vi "test_json_decode.vi"() -> (0 "error out":errorcluster, 3 "all_passed":bool)   [LabVIEW 2019]
panel:
  out "passed":bool[](array[boolean])
  out "values":T1(array[cluster])
  in  "test_cases":T2(array[cluster])
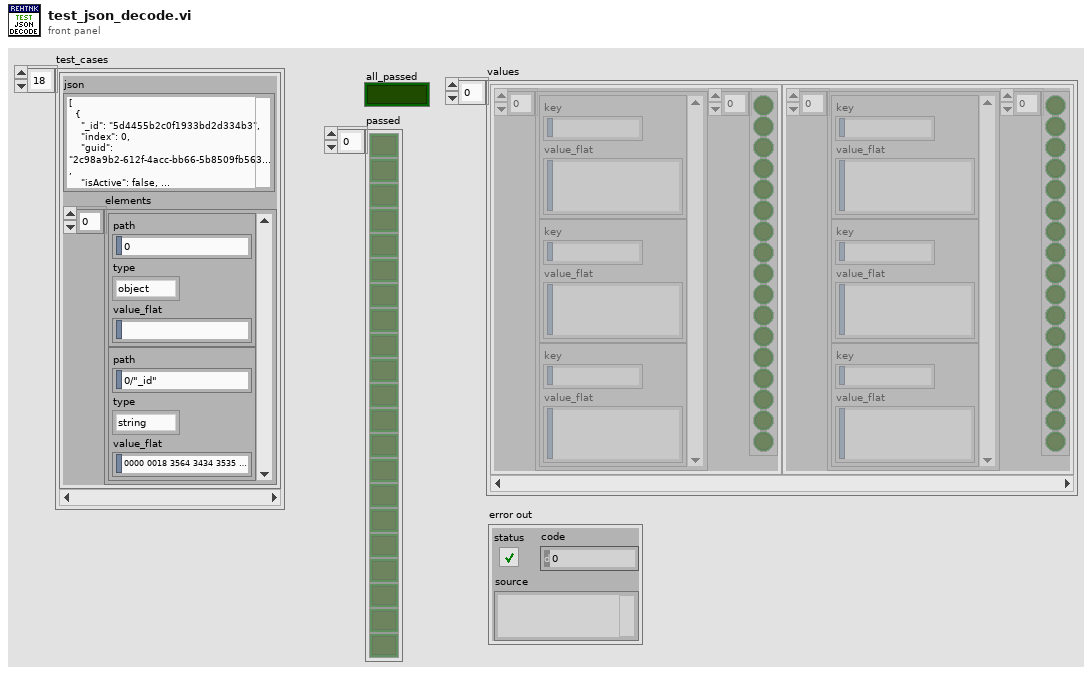
[diagram p1: front panel]
types:
  T1 = cluster{cluster{"key":string, "value_flat":string}[], bool[]}[]
  T2 = cluster{"json":string, "elements":cluster{"path":string, "type":enum8{"null", "bool", "int", "uint", "float", "string", "array", "object"}, "value_flat":string}[]}[]
  T3 = cluster{"path":string, "type":enum8{"null", "bool", "int", "uint", "float", "string", "array", "object"}, "value":variant}[]
  T4 = cluster{"path":string, "type":enum8{"null", "bool", "int", "uint", "float", "string", "array", "object"}, "value_flat":string}[]
  T5 = cluster{"path":string, "type":enum8{"null", "bool", "int", "uint", "float", "string", "array", "object"}, "value":variant}
  T6 = cluster{"path":string, "type":enum8{"null", "bool", "int", "uint", "float", "string", "array", "object"}, "value_flat":string}
  T7 = enum8{"null", "bool", "int", "uint", "float", "string", "array", "object"}
  T8 = cluster{cluster{"key":string, "value_flat":string}[], bool[]}
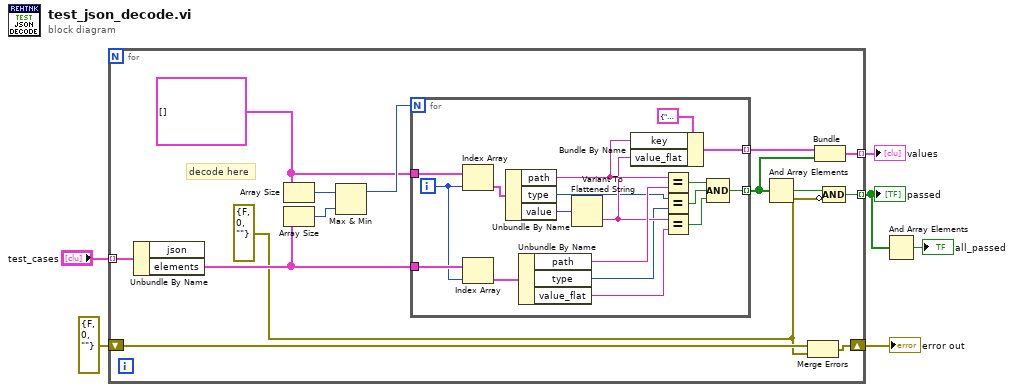
[diagram p0: block diagram]
diagram:
  n1 = for {
    tunnel: "test_cases" -> [w20] mode=indexing
    tunnel: [w14] -> w5 mode=indexing
    tunnel: [w11] -> w4 mode=indexing
    shift-right: [w10] -> w1
    shift-left: errorcluster {"status"=FALSE, "code"=0, "source"=""} ("error out") -> [w9]
    w7 = errorcluster {"status"=FALSE, "code"=0, "source"=""} ("error out")
    w8 = T3 [] ("elements")
    # "decode here"
    n2 = Unbundle By Name(w20) -> ("elements"=w19:T4)  [unwired: 1 out]
    n3 = Array Size(array=w8) -> (size(s)=w18:i32)
    n4 = Array Size(array=w19) -> (size(s)=w17:i32)
    n5 = Max & Min(x=w18, y=w17) -> (max(x,y)=w16:i32)  [unwired: 1 out]
    n6 = for {
      N: w16 -> [_]
      tunnel: w8 -> [w38]
      tunnel: w19 -> [w37]
      tunnel: [w29] -> w15 mode=indexing
      tunnel: [w24] -> w13 mode=indexing
      i -> [w36]
      n7 = Index Array(array=w38, index=w36) -> (element=w35:T5)
      n8 = Index Array(array=w37, index=w36) -> (element=w34:T6)
      n9 = Unbundle By Name(w35) -> ("path"=w30:string, "type"=w23:T7, "value"=w33:variant)
      n10 = Unbundle By Name(w34) -> ("path"=w32:string, "type"=w22:T7, "value_flat"=w27:string)
      n11 = Variant To Flattened String(Variant=w33) -> (data string=w28:string)  [unwired: 1 out]
      n12 = Bundle By Name(cluster=cluster{"key":string, "value_flat":string} {"key"="", "value_flat"=""} ("element"), "key"=w30, "value_flat"=w28) -> (w29:cluster{"key":string, "value_flat":string})
      n13 = Equal?(x=w30, y=w32) -> (x = y?=w25:bool)
      n14 = Equal?(x=w23, y=w22) -> (x = y?=w21:bool)
      n15 = Equal?(x=w28, y=w27) -> (x = y?=w26:bool)
      n16 = Compound Arithmetic op=AND(w25, w21, w26) -> (w24:bool)
    }
    n17 = And Array Elements(Boolean array=w13) -> (logical AND=w12:bool)
    n18 = Merge Errors(w9, w7) -> (w10:errorcluster)
    n19 = Bundle(w15, w13) -> (w14:T8)  [unwired: 1 in]
    n20 = Compound Arithmetic op=AND(w12, invert w7) -> (w11:bool)
  }
  "values" <- w5
  "passed" <- w4
  "error out" <- w1
  n21 = And Array Elements(Boolean array=w4) -> (logical AND=→"all_passed":bool)
